vi "filter.configuration.vi"(10 "Cluster":T13, 11 "filter.data in":T1 {"memory.command"."order.slot.value"."Quantity" format="%016x"; "memory.command"."order.slot.value"."OrderId" format="%016x"; "memory.command"."ticker.slot.value"."Symbol" format="%016x"; "Scratch"."OrderId" format="%016x"}) -> (2 "Boolean":bool, 3 "filter.data out":T1 {"memory.command"."order.slot.value"."Quantity" format="%016x"; "memory.command"."order.slot.value"."OrderId" format="%016x"; "memory.command"."ticker.slot.value"."Symbol" format="%016x"; "Scratch"."OrderId" format="%016x"})   [LabVIEW 2020]
uses:
  filter.data.ctl
  filter.states.ctl
  filter.debug.ctl
  filter.debug.slot.ctl
  filter.data.scratch.ctl
  builds/fpganow.common/orderbook.command.ctl
  builds/fpganow.common/orderbook.command.type.ctl
  filter.memory.command.ctl
  ticker.slot.ctl
  order.slot.ctl
  filter.getstate.ctl
  filter.getstate.slot.ctl
  builds/fpganow.common/fpganow.common.fpga.lvlib
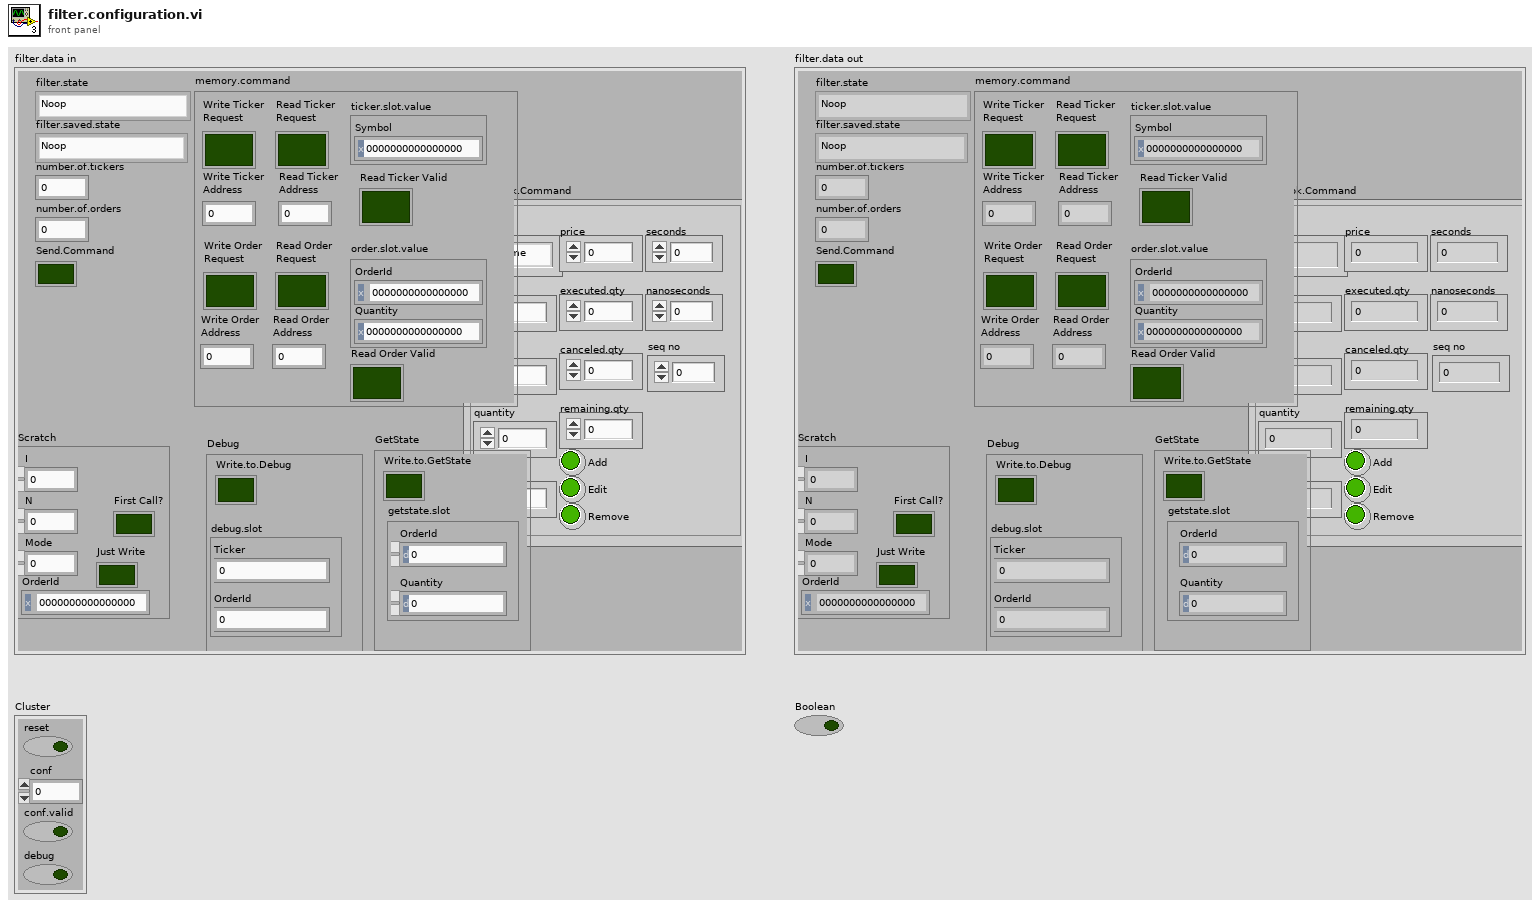
[diagram p1: front panel]
types:
  T1 = typedef "filter.data.ctl" = cluster{"filter.state":T2, "Debug":T3, "number.of.tickers":u32, "number.of.orders":u32, "filter.saved.state":T2, "Scratch":T5, "OrderBook.Command":T6, "Send.Command":bool, "memory.command":T8, "GetState":T11}
  T2 = typedef "filter.states.ctl" = enum16{"Noop", "Reset", "Debug", "Configuration", "Get.State", "Wait.for.Command", "Filter.Add", "Filter.Other", "Insert.Order", "Delete Order"}
  T3 = typedef "filter.debug.ctl" = cluster{"Write.to.Debug":bool, "debug.slot":T4}
  T4 = typedef "filter.debug.slot.ctl" = cluster{"Ticker":u64, "OrderId":u64}
  T5 = typedef "filter.data.scratch.ctl" = cluster{"I":u32, "N":u32, "Mode":u32, "OrderId":u64, "First Call?":bool, "Just Write":bool}
  T6 = typedef "fpganow.common.fpga.lvlib/orderbook.command.ctl" = cluster{"type":T7, "side":u8, "orderId ":u64, "quantity":u32, "symbol":u64, "price":u64, "executed.qty":u32, "canceled.qty":u32, "remaining.qty":u32, "seconds":u64, "nanoseconds":u64, "Add":bool, "Edit":bool, "Remove":bool, "seq no":u32}
  T7 = typedef "fpganow.common.fpga.lvlib/orderbook.command.type.ctl" = enum8{"Time", "AddOrder", "OrderExecuted", "OrderExecutedAtPrice", "ReduceSize", "ModifyOrder", "DeleteOrder", "Get.Everything", "Get.All.Orders", "Get.Top"}
  T8 = typedef "filter.memory.command.ctl" = cluster{"ticker.slot.value":T9, "order.slot.value":T10, "Write Ticker\nAddress":u32, "Write Ticker\nRequest":bool, "Read Ticker\nRequest":bool, "Read Ticker\nAddress":u32, "Read Ticker Valid":bool, "Write Order\nAddress":u32, "Write Order\nRequest":bool, "Read Order\nRequest":bool, "Read Order\nAddress":u32, "Read Order Valid":bool}
  T9 = typedef "ticker.slot.ctl" = cluster{"Symbol":u64}
  T10 = typedef "order.slot.ctl" = cluster{"OrderId":u64, "Quantity":u64}
  T11 = typedef "filter.getstate.ctl" = cluster{"Write.to.GetState":bool, "getstate.slot":T12}
  T12 = typedef "filter.getstate.slot.ctl" = cluster{"OrderId":u64, "Quantity":u64}
  T13 = cluster{"reset":bool, "conf":u64, "conf.valid":bool, "debug":bool}
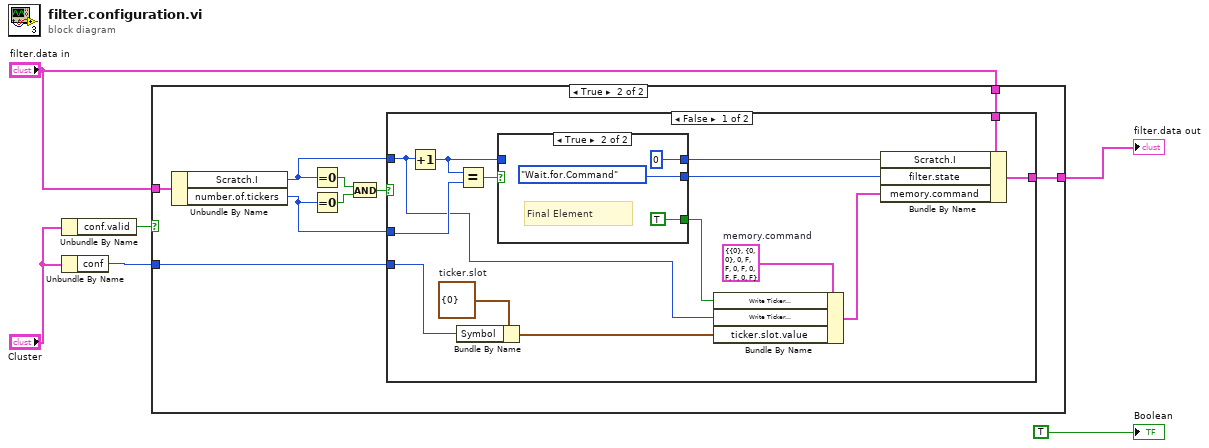
[diagram p0: block diagram]
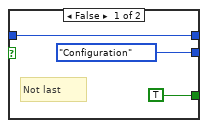
[diagram p3: hidden frame]
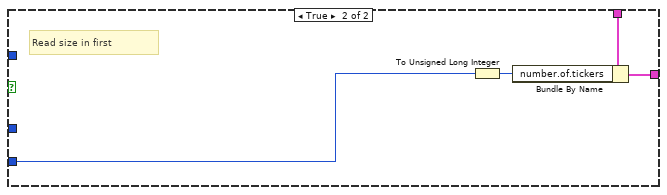
[diagram p4: hidden frame]
diagram:
  n1 = Unbundle By Name("Cluster") -> ("conf.valid"=w1:bool)
  n2 = Unbundle By Name("Cluster") -> ("conf"=w5:u64)
  n3 = case shown="True" w1 {
    tunnel: [w7 w12] -> w2
    tunnel: "filter.data in" -> [w7 w11]
    tunnel: "filter.data in" -> [_ w16]
    tunnel: w5 -> [_ w10]
    frame False {
      # "Noop"
    }
    frame True {
      n4 = Unbundle By Name(w16) -> ("Scratch.I"=w9:u32, "number.of.tickers"=w8:u32)
      n5 = Equal To 0?(x=w9) -> (x = 0?=w15:bool)
      n6 = Equal To 0?(x=w8) -> (x = 0?=w14:bool)
      n7 = And(x=w15, y=w14) -> (x .and. y?=w13:bool)
      n8 = case shown="False" w13 {
        tunnel: [w27 w37] -> w12
        tunnel: w11 -> [w28 w39]
        tunnel: w10 -> [w20 w40]
        tunnel: w9 -> [w18 _]
        tunnel: w8 -> [w30 _]
        frame False {
          w23 = T9 {"Symbol"=0}  # ticker.slot
          w24 = T8 {"ticker.slot.value"={"Symbol"=0}, "order.slot.value"={"OrderId"=0, "Quantity"=0}, "Write Ticker\nAddress"=0, "Write Ticker\nRequest"=FALSE, "Read Ticker\nRequest"=FALSE, "Read Ticker\nAddress"=0, "Read Ticker Valid"=FALSE, "Write Order\nAddress"=0, "Write Order\nRequest"=FALSE, "Read Order\nRequest"=FALSE, "Read Order\nAddress"=0, "Read Order Valid"=FALSE}  # memory.command
          n9 = Increment(x=w18) -> (x+1=w25:u32)
          n10 = Bundle By Name(cluster=w23, "Symbol"=w20) -> (w22:T9)
          n11 = Equal?(x=w25, y=w30) -> (x = y?=w29:bool)
          n12 = case shown="True" w29 {
            tunnel: w25 -> [w32 _]
            tunnel: [w32 u32 0] -> w26
            tunnel: [filter.states."Configuration" ("filter.states") filter.states."Wait.for.Command" ("filter.states")] -> w19
            tunnel: [TRUE ("Write Order\nRequest") TRUE ("Write Order\nRequest")] -> w17
            frame False {
              # "Not last"
            }
            frame True {
              # "Final Element"
            }
          }
          n13 = Bundle By Name(cluster=w24, "Write Ticker\nRequest"=w17, "Write Ticker\nAddress"=w18, "ticker.slot.value"=w22) -> (w21:T8)
          n14 = Bundle By Name(cluster=w28, "Scratch.I"=w26, "filter.state"=w19, "memory.command"=w21) -> (w27:T1)
        }
        frame True {
          # "Read size in first"
          n15 = To Unsigned Long Integer(number=w40) -> (unsigned 32bit integer=w38:u32)
          n16 = Bundle By Name(cluster=w39, "number.of.tickers"=w38) -> (w37:T1)
        }
      }
    }
  }
  "filter.data out" <- w2
  "Boolean" <- TRUE
